vi "SGL Wordswap.vi"(1 "x":sgl) -> (0 "*(type *) &x":sgl)   [LabVIEW 2020]
doc: "This VI does a wordswap of SGL datatype to allow it to work with different representations."
panel:
  in  "x 2":sgl
  in  "Array":i8[](array[numeric])
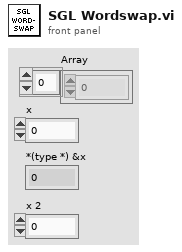
[diagram p1: front panel]
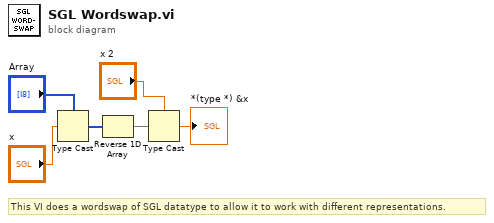
[diagram p0: block diagram]
diagram:
  # "This VI does a wordswap of SGL datatype to allow it to work with different representations."
  n1 = Type Cast(type="Array", x="x") -> (*(type *) &x=w4:i8[])
  n2 = Reverse 1D Array(array=w4) -> (reversed array=w3:i8[])
  n3 = Type Cast(type="x 2", x=w3) -> (*(type *) &x=→"*(type *) &x":sgl)
